vi "Constructor.vi"(8 "error in (no error)":errorcluster, 11 "Class in":refnum<class>) -> (0 "error out":errorcluster, 3 "Singleton out":refnum<class "Provider.lvclass">)   [LabVIEW 2020, in "Provider.lvlib" / "Provider.lvclass"]
uses:
  Provider.lvclass
  Provider.lvclass/Provider.ctl
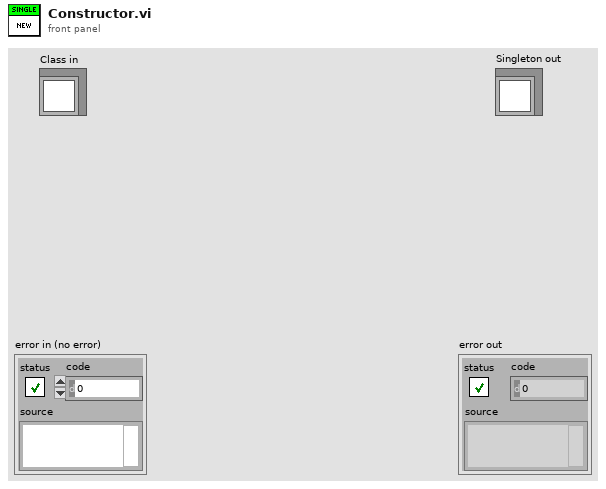
[diagram p1: front panel]
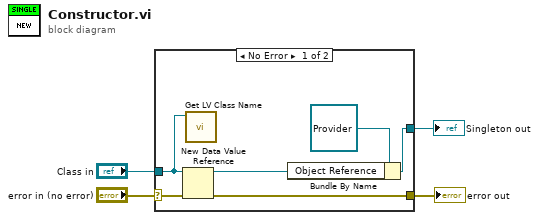
[diagram p0: block diagram]
diagram:
  n1 = case shown="No Error" "error in (no error)" {
    selector: "error in (no error)" -> [w10 w11]
    tunnel: [w9 w11] -> w3
    tunnel: "Class in" -> [w5 _]
    tunnel: [w8 _] -> w1
    frame No Error {
      n2 = New Data Value Reference(data value=w5, error in=w10) -> (data value reference=w6:refnum<data-value>, error out=w9:errorcluster)
      n3 = call <vilib>:"Get LV Class Name.vi"("object"=w5) -> ()  [unwired: 9 in, 2 out]
      n4 = Bundle By Name(cluster=refnum<class "Provider.lvclass"> refnum ("Singleton out"), "Object Reference"=w6) -> (w8:refnum<class "Provider.lvclass">)
    }
    frame Error {
    }
  }
  "error out" <- w3
  "Singleton out" <- w1
